vi "Launcher.vi"(8 "error in (no error)":errorcluster, 10 "Log Class":refnum<class "Build_Javier_Lopez_lib_Configuration_Filejson class.lvclass">, 11 "Module Meta in":refnum<class "Version.lvclass">) -> (0 "error out":errorcluster)   [LabVIEW 2021, in "Version.lvclass"]
uses:
  Version.lvclass
  <vilib>/Javier Lopez/Configuration File/Json Element/Build_Javier_Lopez_lib_Configuration_Filejson class.lvclass
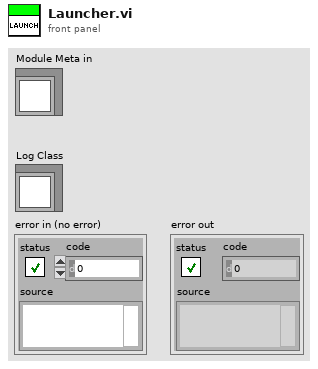
[diagram p1: front panel]
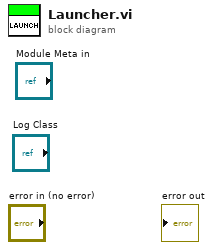
[diagram p0: block diagram]
diagram:
